vi "get vi name.vi"(11 "library.lvlib:name.vi":string) -> (3 "vi name":string)   [LabVIEW 2017]
doc: "Converts VI name in the format 'library.lvlib:name.vi' to 'name'\n____________________________________________\nDIPC 692 Daemon API 10.0.0.1\nSam Tee - Dyson Technology Ltd\nCopyright (c) 2024, Dyson Technology Ltd"
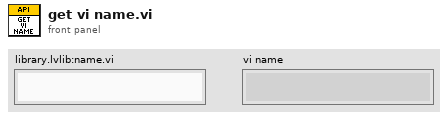
[diagram p1: front panel]
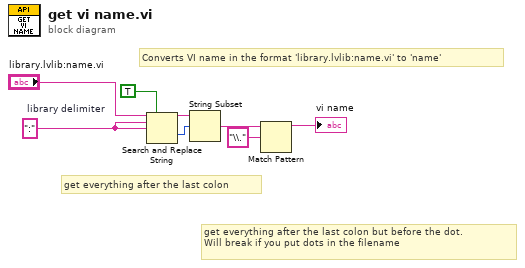
[diagram p0: block diagram]
diagram:
  w8 = ":"  # library delimiter
  # "Converts VI name in the format 'library.lvlib:name.vi' to 'name'"
  # "get everything after the last colon but before the dot.\nWill break if you put dots in the filename"
  # "get everything after the last colon"
  n1 = Search and Replace String(replace all?=TRUE ("replace all? (F)"), input string="library.lvlib:name.vi", search string=w8, replace string=w8) -> (result string=w5:string, offset past replacement=w4:i32)  [unwired: 4 in, 2 out]
  n2 = String Subset(string=w5, offset (0)=w4) -> (substring=w3:string)  [unwired: 1 in]
  n3 = Match Pattern(string=w3, regular expression="\\.") -> (before substring=→"vi name":string)  [unwired: 1 in, 3 out]
